vi "MQTTParse.vi"(0 "topic":string, 1 "Input message":T2) -> (4 "Success?":bool, 5 "Double":dbl, 6 "String":string)   [LabVIEW 2017]
uses:
  <vilib>/daq.io/MQTT LabVIEW Client/Controls/MessageType.ctl
  <vilib>/daq.io/MQTT LabVIEW Client/MQTT_Functions.lvlib
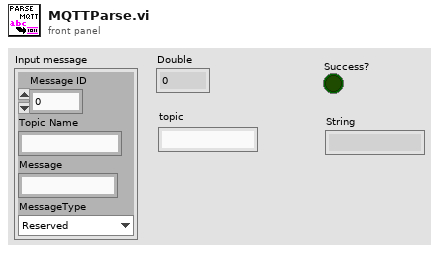
[diagram p1: front panel]
types:
  T1 = typedef "MQTT_Functions.lvlib/MessageType.ctl" = enum32{"Reserved", "CONNECT", "CONNACK", "PUBLISH", "PUBACK", "PUBREC", "PUBREL", "PUBCOMP", "SUBSCRIBE", "SUBACK", "UNSUBSCRIBE", "UNSUBACK", "PINGREQ", "PINGRESP", "DISCONNECT", "Reserved2"}
  T2 = cluster{"Message ID":u16, "Topic Name":string, "Message":string, "MessageType":T1}
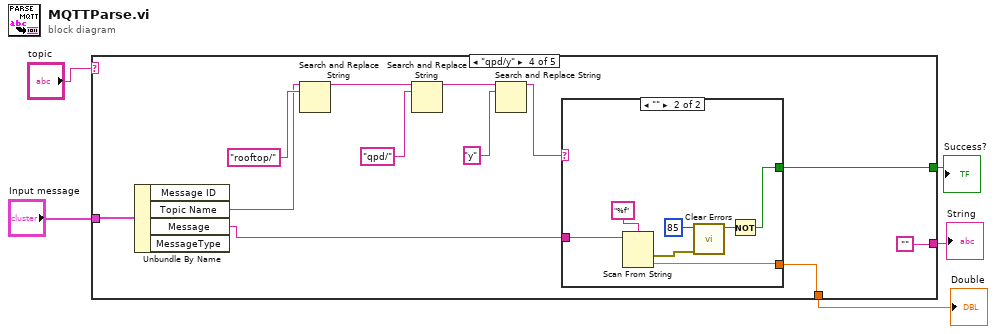
[diagram p0: block diagram]
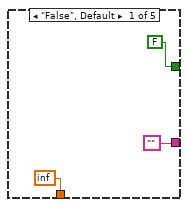
[diagram p2: hidden frame]
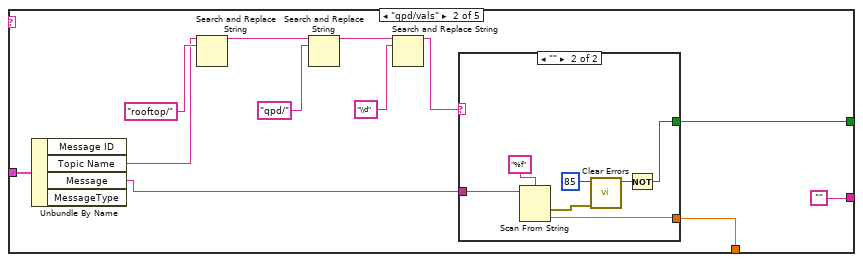
[diagram p3: hidden frame]
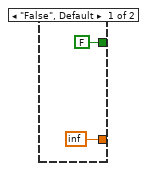
[diagram p4: hidden frame]
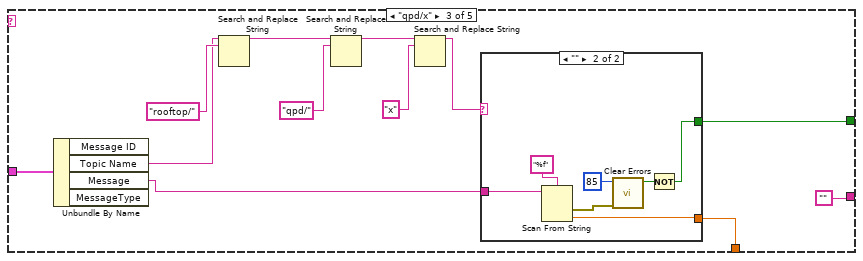
[diagram p5: hidden frame]
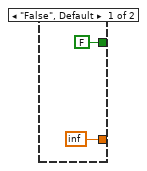
[diagram p6: hidden frame]
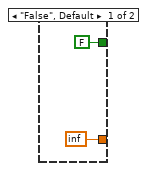
[diagram p7: hidden frame]
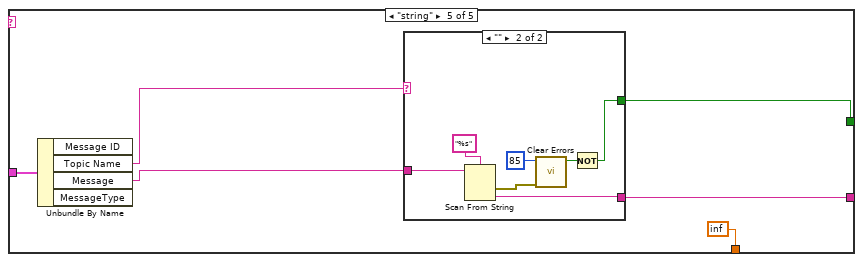
[diagram p8: hidden frame]
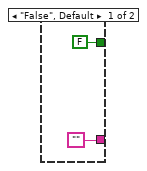
[diagram p9: hidden frame]
diagram:
  n1 = case shown="\"qpd/y\"" "topic" {
    tunnel: "Input message" -> [_ w20 w33 w54 w76]
    tunnel: [FALSE w11 w32 w51 w77] -> w3
    tunnel: ["" "" "" "" w73] -> w2
    tunnel: [inf w10 w31 w53 inf] -> w1
    frame "False", Default {
    }
    frame "qpd/vals" {
      n2 = Unbundle By Name(w20) -> ("Topic Name"=w12:string, "Message"=w13:string)  [unwired: 2 out]
      n3 = Search and Replace String(input string=w12, search string="rooftop/" ("regular expression")) -> (result string=w17:string)  [unwired: 6 in, 3 out]
      n4 = Search and Replace String(input string=w17, search string="qpd/" ("regular expression")) -> (result string=w16:string)  [unwired: 6 in, 3 out]
      n5 = Search and Replace String(input string=w16, search string="\\d" ("regular expression")) -> (result string=w14:string)  [unwired: 6 in, 3 out]
      n6 = case shown="\"\"" w14 {
        tunnel: w13 -> [_ w26]
        tunnel: [inf w25] -> w10
        tunnel: [FALSE w24] -> w11
        frame "False", Default {
        }
        frame "" {
          n7 = Scan From String(format string="%f", input string=w26) -> (error out=w29:errorcluster, output 1=w25:dbl)  [unwired: 3 in, 2 out]
          n8 = call <vilib>:"Clear Errors.vi"("error in (no error)"=w29, "specific error code to clear (0: all)"=85) -> ("specific error cleared?"=w27:bool)  [unwired: 4 in, 1 out]
          n9 = Not(x=w27) -> (.not. x?=w24:bool)
        }
      }
    }
    frame "qpd/x" {
      n10 = Unbundle By Name(w33) -> ("Topic Name"=w34:string, "Message"=w35:string)  [unwired: 2 out]
      n11 = Search and Replace String(input string=w34, search string="rooftop/" ("regular expression")) -> (result string=w39:string)  [unwired: 6 in, 3 out]
      n12 = Search and Replace String(input string=w39, search string="qpd/" ("regular expression")) -> (result string=w38:string)  [unwired: 6 in, 3 out]
      n13 = Search and Replace String(input string=w38, search string="x" ("regular expression")) -> (result string=w36:string)  [unwired: 6 in, 3 out]
      n14 = case shown="\"\"" w36 {
        tunnel: w35 -> [_ w47]
        tunnel: [inf w46] -> w31
        tunnel: [FALSE w45] -> w32
        frame "False", Default {
        }
        frame "" {
          n15 = Scan From String(format string="%f", input string=w47) -> (error out=w50:errorcluster, output 1=w46:dbl)  [unwired: 3 in, 2 out]
          n16 = call <vilib>:"Clear Errors.vi"("error in (no error)"=w50, "specific error code to clear (0: all)"=85) -> ("specific error cleared?"=w48:bool)  [unwired: 4 in, 1 out]
          n17 = Not(x=w48) -> (.not. x?=w45:bool)
        }
      }
    }
    frame "qpd/y" {
      n18 = Unbundle By Name(w54) -> ("Topic Name"=w55:string, "Message"=w56:string)  [unwired: 2 out]
      n19 = Search and Replace String(input string=w55, search string="rooftop/" ("regular expression")) -> (result string=w60:string)  [unwired: 6 in, 3 out]
      n20 = Search and Replace String(input string=w60, search string="qpd/" ("regular expression")) -> (result string=w59:string)  [unwired: 6 in, 3 out]
      n21 = Search and Replace String(input string=w59, search string="y" ("regular expression")) -> (result string=w57:string)  [unwired: 6 in, 3 out]
      n22 = case shown="\"\"" w57 {
        tunnel: w56 -> [_ w68]
        tunnel: [inf w67] -> w53
        tunnel: [FALSE w66] -> w51
        frame "False", Default {
        }
        frame "" {
          n23 = Scan From String(format string="%f", input string=w68) -> (error out=w71:errorcluster, output 1=w67:dbl)  [unwired: 3 in, 2 out]
          n24 = call <vilib>:"Clear Errors.vi"("error in (no error)"=w71, "specific error code to clear (0: all)"=85) -> ("specific error cleared?"=w69:bool)  [unwired: 4 in, 1 out]
          n25 = Not(x=w69) -> (.not. x?=w66:bool)
        }
      }
    }
    frame "string" {
      n26 = Unbundle By Name(w76) -> ("Topic Name"=w75:string, "Message"=w74:string)  [unwired: 2 out]
      n27 = case shown="\"\"" w75 {
        tunnel: w74 -> [_ w83]
        tunnel: [FALSE w82] -> w77
        tunnel: ["" w80] -> w73
        frame "False", Default {
        }
        frame "" {
          n28 = Scan From String(format string="%s", input string=w83) -> (error out=w86:errorcluster, output 1=w80:string)  [unwired: 3 in, 2 out]
          n29 = call <vilib>:"Clear Errors.vi"("error in (no error)"=w86, "specific error code to clear (0: all)"=85) -> ("specific error cleared?"=w84:bool)  [unwired: 4 in, 1 out]
          n30 = Not(x=w84) -> (.not. x?=w82:bool)
        }
      }
    }
  }
  "Success?" <- w3
  "String" <- w2
  "Double" <- w1
